vi "Set LVClass Path.vi"(10 "LVClass Path":path, 11 "Manifestation Writer in":refnum<class "Manifestation Writer.lvclass">) -> (3 "Manifestation Writer out":refnum<class "Manifestation Writer.lvclass">)   [LabVIEW 2013, in "Manifestation Writer.lvclass"]
doc: "Copyright (c) 2016 Sze Howe Koh\n\nThis Source Code Form is subject to the terms of the Mozilla Public License, v. 2.0. If a copy of the MPL was not distributed with this file, You can obtain one at http://mozilla.org/MPL/2.0/."
uses:
  Manifestation Writer.lvclass
  Manifestation Writer.lvclass/Manifestation Writer.ctl
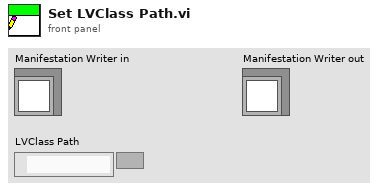
[diagram p1: front panel]
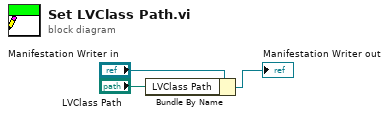
[diagram p0: block diagram]
diagram:
  n1 = Bundle By Name(cluster="Manifestation Writer in", "LVClass Path"="LVClass Path") -> (→"Manifestation Writer out":refnum<class "Manifestation Writer.lvclass">)
